vi "Send Value to Caller.vi"(8 "error in (no error)":errorcluster, 11 "H3611i Actor in":refnum<class "H3611i Actor.lvclass">) -> (0 "error out":errorcluster, 3 "H3611i Actor out":refnum<class "H3611i Actor.lvclass">)   [LabVIEW 2017]
uses:
  H3611i Actor.lvclass
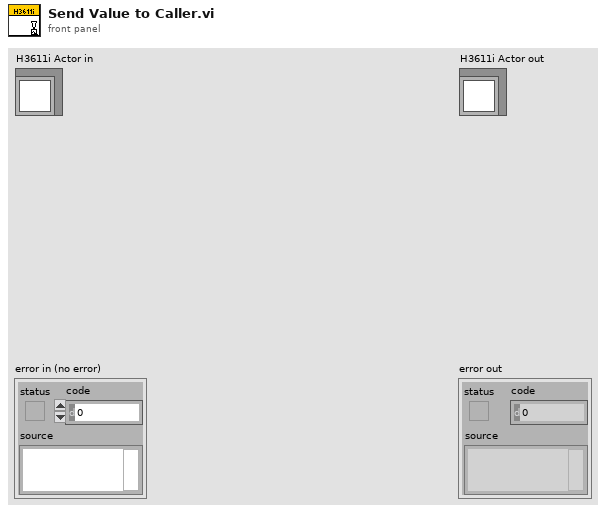
[diagram p1: front panel]
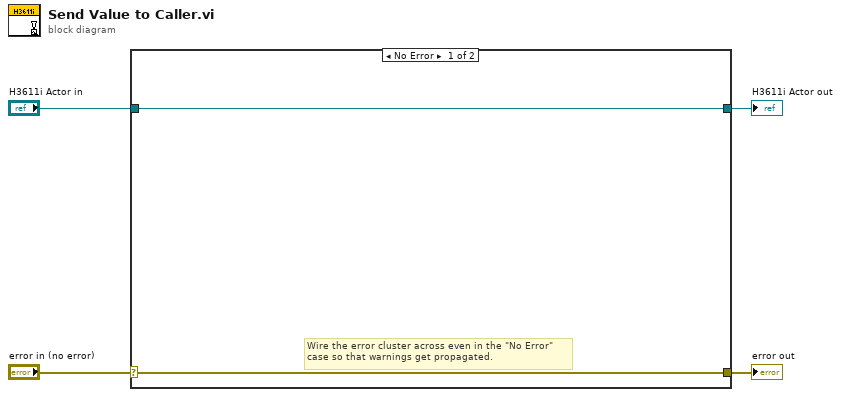
[diagram p0: block diagram]
diagram:
  n1 = case shown="No Error" "error in (no error)" {
    selector: "error in (no error)" -> [w5 w8]
    tunnel: [w5 w8] -> w3
    tunnel: [w6 w7] -> w1
    tunnel: "H3611i Actor in" -> [w6 w7]
    frame No Error {
      # "Wire the error cluster across even in the \"No Error\"\ncase so that warnings get propagated."
    }
    frame Error {
    }
  }
  "error out" <- w3
  "H3611i Actor out" <- w1
